vi "RTS Station 5 Doors.vi"(0 "All Door Opener Ctrl in":T11={"Station 1"={"Station Freezer"={"Time Count (s)"=0.0, "Status"="", "Door State"=FALSE, "Delay"=FALSE, "Chamber 1-1"=[], "Index"=0, "Delay Status"=""}, "Station Cab"={"Time Count (s)"=0.0, "Status"="", "Door State"=FALSE, "Delay"=FALSE, "Chamber 1-1"=[], "Index"=0, "Delay Status"=""}, "Station Slide"={"Time Count (s)"=0.0, "Status"="", "Door State"=FALSE, "Delay"=FALSE, "Chamber 1-1"=[], "Index"=0, "Delay Status"=""}, "1st Complete"=FALSE, "2nd Complete"=FALSE, "3rd Complete"=FALSE}, "Station 2"={"Station Freezer"={"Time Count (s)"=0.0, "Status"="", "Door State"=FALSE, "Delay"=FALSE, "Chamber 1-1"=[], "Index"=0, "Delay Status"=""}, "Station Cab"={"Time Count (s)"=0.0, "Status"="", "Door State"=FALSE, "Delay"=FALSE, "Chamber 1-1"=[], "Index"=0, "Delay Status"=""}, "Station Slide"={"Time Count (s)"=0.0, "Status"="", "Door State"=FALSE, "Delay"=FALSE, "Chamber 1-1"=[], "Index"=0, "Delay Status"=""}, "1st Complete"=FALSE, "2nd Complete"=FALSE, "3rd Complete"=FALSE}, "Station 3"={"Station Freezer"={"Time Count (s)"=0.0, "Status"="", "Door State"=FALSE, "Delay"=FALSE, "Chamber 1-1"=[], "Index"=0, "Delay Status"=""}, "Station Cab"={"Time Count (s)"=0.0, "Status"="", "Door State"=FALSE, "Delay"=FALSE, "Chamber 1-1"=[], "Index"=0, "Delay Status"=""}, "Station Slide"={"Time Count (s)"=0.0, "Status"="", "Door State"=FALSE, "Delay"=FALSE, "Chamber 1-1"=[], "Index"=0, "Delay Status"=""}, "1st Complete"=FALSE, "2nd Complete"=FALSE, "3rd Complete"=FALSE}, "Station 4"={"Station Freezer"={"Time Count (s)"=0.0, "Status"="", "Door State"=FALSE, "Delay"=FALSE, "Chamber 1-1"=[], "Index"=0, "Delay Status"=""}, "Station Cab"={"Time Count (s)"=0.0, "Status"="", "Door State"=FALSE, "Delay"=FALSE, "Chamber 1-1"=[], "Index"=0, "Delay Status"=""}, "Station Slide"={"Time Count (s)"=0.0, "Status"="", "Door State"=FALSE, "Delay"=FALSE, "Chamber 1-1"=[], "Index"=0, "Delay Status"=""}, "1st Complete"=FALSE, "2nd Complete"=FALSE, "3rd Complete"=FALSE}, "Station 5"={"Station Freezer"={"Time Count (s)"=0.0, "Status"="", "Door State"=FALSE, "Delay"=TRUE, "Chamber 1-1"=[], "Index"=0, "Delay Status"=""}, "Station Cab"={"Time Count (s)"=0.0, "Status"="", "Door State"=FALSE, "Delay"=TRUE, "Chamber 1-1"=[], "Index"=0, "Delay Status"=""}, "Station Slide"={"Time Count (s)"=0.0, "Status"="", "Door State"=FALSE, "Delay"=TRUE, "Chamber 1-1"=[], "Index"=0, "Delay Status"=""}, "1st Complete"=FALSE, "2nd Complete"=FALSE, "3rd Complete"=FALSE}, "Station 6"={"Station Freezer"={"Time Count (s)"=0.0, "Status"="", "Door State"=FALSE, "Delay"=TRUE, "Chamber 1-1"=[], "Index"=0, "Delay Status"=""}, "Station Cab"={"Time Count (s)"=0.0, "Status"="", "Door State"=FALSE, "Delay"=TRUE, "Chamber 1-1"=[], "Index"=0, "Delay Status"=""}, "Station Slide"={"Time Count (s)"=0.0, "Status"="", "Door State"=FALSE, "Delay"=TRUE, "Chamber 1-1"=[], "Index"=0, "Delay Status"=""}, "1st Complete"=FALSE, "2nd Complete"=FALSE, "3rd Complete"=FALSE}, "Station 7"={"Station Freezer"={"Time Count (s)"=0.0, "Status"="", "Door State"=FALSE, "Delay"=TRUE, "Chamber 1-1"=[], "Index"=0, "Delay Status"=""}, "Station Cab"={"Time Count (s)"=0.0, "Status"="", "Door State"=FALSE, "Delay"=TRUE, "Chamber 1-1"=[], "Index"=0, "Delay Status"=""}, "Station Slide"={"Time Count (s)"=0.0, "Status"="", "Door State"=FALSE, "Delay"=TRUE, "Chamber 1-1"=[], "Index"=0, "Delay Status"=""}, "1st Complete"=FALSE, "2nd Complete"=FALSE, "3rd Complete"=FALSE}, "Station 8"={"Station Freezer"={"Time Count (s)"=0.0, "Status"="", "Door State"=FALSE, "Delay"=TRUE, "Chamber 1-1"=[], "Index"=0, "Delay Status"=""}, "Station Cab"={"Time Count (s)"=0.0, "Status"="", "Door State"=FALSE, "Delay"=TRUE, "Chamber 1-1"=[], "Index"=0, "Delay Status"=""}, "Station Slide"={"Time Count (s)"=0.0, "Status"="", "Door State"=FALSE, "Delay"=TRUE, "Chamber 1-1"=[], "Index"=0, "Delay Status"=""}, "1st Complete"=FALSE, "2nd Complete"=FALSE, "3rd Complete"=FALSE}} {"Station 8"."Station Slide"."Chamber 1-1"."Start Time" format="%<%X\n%x>T"; "Station 8"."Station Slide"."Chamber 1-1"."End Time" format="%<%X\n%x>T"; "Station 8"."Station Slide"."Time Count (s)" format="%.2f"; "Station 8"."Station Cab"."Chamber 1-1"."Start Time" format="%<%X\n%x>T"; "Station 8"."Station Cab"."Chamber 1-1"."End Time" format="%<%X\n%x>T"; "Station 8"."Station Cab"."Time Count (s)" format="%.2f"; "Station 8"."Station Freezer"."Chamber 1-1"."Start Time" format="%<%X\n%x>T"; "Station 8"."Station Freezer"."Chamber 1-1"."End Time" format="%<%X\n%x>T"; "Station 8"."Station Freezer"."Time Count (s)" format="%.2f"; "Station 7"."Station Slide"."Chamber 1-1"."Start Time" format="%<%X\n%x>T"; "Station 7"."Station Slide"."Chamber 1-1"."End Time" format="%<%X\n%x>T"; "Station 7"."Station Slide"."Time Count (s)" format="%.2f"; "Station 7"."Station Cab"."Chamber 1-1"."Start Time" format="%<%X\n%x>T"; "Station 7"."Station Cab"."Chamber 1-1"."End Time" format="%<%X\n%x>T"; "Station 7"."Station Cab"."Time Count (s)" format="%.2f"; "Station 7"."Station Freezer"."Chamber 1-1"."Start Time" format="%<%X\n%x>T"; "Station 7"."Station Freezer"."Chamber 1-1"."End Time" format="%<%X\n%x>T"; "Station 7"."Station Freezer"."Time Count (s)" format="%.2f"; "Station 6"."Station Slide"."Chamber 1-1"."Start Time" format="%<%X\n%x>T"; "Station 6"."Station Slide"."Chamber 1-1"."End Time" format="%<%X\n%x>T"; "Station 6"."Station Slide"."Time Count (s)" format="%.2f"; "Station 6"."Station Cab"."Chamber 1-1"."Start Time" format="%<%X\n%x>T"; "Station 6"."Station Cab"."Chamber 1-1"."End Time" format="%<%X\n%x>T"; "Station 6"."Station Cab"."Time Count (s)" format="%.2f"; "Station 6"."Station Freezer"."Chamber 1-1"."Start Time" format="%<%X\n%x>T"; "Station 6"."Station Freezer"."Chamber 1-1"."End Time" format="%<%X\n%x>T"; "Station 6"."Station Freezer"."Time Count (s)" format="%.2f"; "Station 5"."Station Slide"."Chamber 1-1"."Start Time" format="%<%X\n%x>T"; "Station 5"."Station Slide"."Chamber 1-1"."End Time" format="%<%X\n%x>T"; "Station 5"."Station Slide"."Time Count (s)" format="%.2f"; "Station 5"."Station Cab"."Chamber 1-1"."Start Time" format="%<%X\n%x>T"; "Station 5"."Station Cab"."Chamber 1-1"."End Time" format="%<%X\n%x>T"; "Station 5"."Station Cab"."Time Count (s)" format="%.2f"; "Station 5"."Station Freezer"."Chamber 1-1"."Start Time" format="%<%X\n%x>T"; "Station 5"."Station Freezer"."Chamber 1-1"."End Time" format="%<%X\n%x>T"; "Station 5"."Station Freezer"."Time Count (s)" format="%.2f"; "Station 4"."Station Slide"."Chamber 1-1"."Start Time" format="%<%X\n%x>T"; "Station 4"."Station Slide"."Chamber 1-1"."End Time" format="%<%X\n%x>T"; "Station 4"."Station Slide"."Time Count (s)" format="%.2f"; "Station 4"."Station Cab"."Chamber 1-1"."Start Time" format="%<%X\n%x>T"; "Station 4"."Station Cab"."Chamber 1-1"."End Time" format="%<%X\n%x>T"; "Station 4"."Station Cab"."Time Count (s)" format="%.2f"; "Station 4"."Station Freezer"."Chamber 1-1"."Start Time" format="%<%X\n%x>T"; "Station 4"."Station Freezer"."Chamber 1-1"."End Time" format="%<%X\n%x>T"; "Station 4"."Station Freezer"."Time Count (s)" format="%.2f"; "Station 3"."Station Slide"."Chamber 1-1"."Start Time" format="%<%X\n%x>T"; "Station 3"."Station Slide"."Chamber 1-1"."End Time" format="%<%X\n%x>T"; "Station 3"."Station Slide"."Time Count (s)" format="%.2f"; "Station 3"."Station Cab"."Chamber 1-1"."Start Time" format="%<%X\n%x>T"; "Station 3"."Station Cab"."Chamber 1-1"."End Time" format="%<%X\n%x>T"; "Station 3"."Station Cab"."Time Count (s)" format="%.2f"; "Station 3"."Station Freezer"."Chamber 1-1"."Start Time" format="%<%X\n%x>T"; "Station 3"."Station Freezer"."Chamber 1-1"."End Time" format="%<%X\n%x>T"; "Station 3"."Station Freezer"."Time Count (s)" format="%.2f"; "Station 2"."Station Slide"."Chamber 1-1"."Start Time" format="%<%X\n%x>T"; "Station 2"."Station Slide"."Chamber 1-1"."End Time" format="%<%X\n%x>T"; "Station 2"."Station Slide"."Time Count (s)" format="%.2f"; "Station 2"."Station Cab"."Chamber 1-1"."Start Time" format="%<%X\n%x>T"; "Station 2"."Station Cab"."Chamber 1-1"."End Time" format="%<%X\n%x>T"; "Station 2"."Station Cab"."Time Count (s)" format="%.2f"; "Station 2"."Station Freezer"."Chamber 1-1"."Start Time" format="%<%X\n%x>T"; "Station 2"."Station Freezer"."Chamber 1-1"."End Time" format="%<%X\n%x>T"; "Station 2"."Station Freezer"."Time Count (s)" format="%.2f"; "Station 1"."Station Slide"."Chamber 1-1"."Start Time" format="%<%X\n%x>T"; "Station 1"."Station Slide"."Chamber 1-1"."End Time" format="%<%X\n%x>T"; "Station 1"."Station Slide"."Time Count (s)" format="%.2f"; "Station 1"."Station Cab"."Chamber 1-1"."Start Time" format="%<%X\n%x>T"; "Station 1"."Station Cab"."Chamber 1-1"."End Time" format="%<%X\n%x>T"; "Station 1"."Station Cab"."Time Count (s)" format="%.2f"; "Station 1"."Station Freezer"."Chamber 1-1"."Start Time" format="%<%X\n%x>T"; "Station 1"."Station Freezer"."Chamber 1-1"."End Time" format="%<%X\n%x>T"; "Station 1"."Station Freezer"."Time Count (s)" format="%.2f"}, 1 "Door Output Relays":T10, 5 "Input":refnum<class "Modbus Master.lvclass">, 7 "RTS Config Setup Input":T1, 11 "Error In":errorcluster) -> (4 "All Door Opener Ctrl Output":T11={"Station 1"={"Station Freezer"={"Time Count (s)"=0.0, "Status"="", "Door State"=FALSE, "Delay"=TRUE, "Chamber 1-1"=[], "Index"=0, "Delay Status"=""}, "Station Cab"={"Time Count (s)"=0.0, "Status"="", "Door State"=FALSE, "Delay"=TRUE, "Chamber 1-1"=[], "Index"=0, "Delay Status"=""}, "Station Slide"={"Time Count (s)"=0.0, "Status"="", "Door State"=FALSE, "Delay"=TRUE, "Chamber 1-1"=[], "Index"=0, "Delay Status"=""}, "1st Complete"=TRUE, "2nd Complete"=FALSE, "3rd Complete"=FALSE}, "Station 2"={"Station Freezer"={"Time Count (s)"=0.0, "Status"="", "Door State"=FALSE, "Delay"=TRUE, "Chamber 1-1"=[], "Index"=0, "Delay Status"=""}, "Station Cab"={"Time Count (s)"=0.0, "Status"="", "Door State"=FALSE, "Delay"=TRUE, "Chamber 1-1"=[], "Index"=0, "Delay Status"=""}, "Station Slide"={"Time Count (s)"=0.0, "Status"="", "Door State"=FALSE, "Delay"=TRUE, "Chamber 1-1"=[], "Index"=0, "Delay Status"=""}, "1st Complete"=TRUE, "2nd Complete"=FALSE, "3rd Complete"=FALSE}, "Station 3"={"Station Freezer"={"Time Count (s)"=0.0, "Status"="", "Door State"=FALSE, "Delay"=TRUE, "Chamber 1-1"=[], "Index"=0, "Delay Status"=""}, "Station Cab"={"Time Count (s)"=0.0, "Status"="", "Door State"=FALSE, "Delay"=TRUE, "Chamber 1-1"=[], "Index"=0, "Delay Status"=""}, "Station Slide"={"Time Count (s)"=0.0, "Status"="", "Door State"=FALSE, "Delay"=TRUE, "Chamber 1-1"=[], "Index"=0, "Delay Status"=""}, "1st Complete"=TRUE, "2nd Complete"=FALSE, "3rd Complete"=FALSE}, "Station 4"={"Station Freezer"={"Time Count (s)"=0.0, "Status"="", "Door State"=FALSE, "Delay"=TRUE, "Chamber 1-1"=[], "Index"=0, "Delay Status"=""}, "Station Cab"={"Time Count (s)"=0.0, "Status"="", "Door State"=FALSE, "Delay"=TRUE, "Chamber 1-1"=[], "Index"=0, "Delay Status"=""}, "Station Slide"={"Time Count (s)"=0.0, "Status"="", "Door State"=FALSE, "Delay"=TRUE, "Chamber 1-1"=[], "Index"=0, "Delay Status"=""}, "1st Complete"=TRUE, "2nd Complete"=FALSE, "3rd Complete"=FALSE}, "Station 5"={"Station Freezer"={"Time Count (s)"=0.0, "Status"="", "Door State"=TRUE, "Delay"=TRUE, "Chamber 1-1"=[], "Index"=0, "Delay Status"=""}, "Station Cab"={"Time Count (s)"=0.0, "Status"="", "Door State"=FALSE, "Delay"=TRUE, "Chamber 1-1"=[], "Index"=0, "Delay Status"=""}, "Station Slide"={"Time Count (s)"=0.0, "Status"="", "Door State"=FALSE, "Delay"=TRUE, "Chamber 1-1"=[], "Index"=0, "Delay Status"=""}, "1st Complete"=TRUE, "2nd Complete"=FALSE, "3rd Complete"=FALSE}, "Station 6"={"Station Freezer"={"Time Count (s)"=0.0, "Status"="", "Door State"=FALSE, "Delay"=TRUE, "Chamber 1-1"=[], "Index"=0, "Delay Status"=""}, "Station Cab"={"Time Count (s)"=0.0, "Status"="", "Door State"=FALSE, "Delay"=TRUE, "Chamber 1-1"=[], "Index"=0, "Delay Status"=""}, "Station Slide"={"Time Count (s)"=0.0, "Status"="", "Door State"=FALSE, "Delay"=TRUE, "Chamber 1-1"=[], "Index"=0, "Delay Status"=""}, "1st Complete"=TRUE, "2nd Complete"=FALSE, "3rd Complete"=FALSE}, "Station 7"={"Station Freezer"={"Time Count (s)"=0.0, "Status"="", "Door State"=FALSE, "Delay"=TRUE, "Chamber 1-1"=[], "Index"=0, "Delay Status"=""}, "Station Cab"={"Time Count (s)"=0.0, "Status"="", "Door State"=FALSE, "Delay"=TRUE, "Chamber 1-1"=[], "Index"=0, "Delay Status"=""}, "Station Slide"={"Time Count (s)"=0.0, "Status"="", "Door State"=FALSE, "Delay"=TRUE, "Chamber 1-1"=[], "Index"=0, "Delay Status"=""}, "1st Complete"=TRUE, "2nd Complete"=FALSE, "3rd Complete"=FALSE}, "Station 8"={"Station Freezer"={"Time Count (s)"=0.0, "Status"="", "Door State"=FALSE, "Delay"=TRUE, "Chamber 1-1"=[], "Index"=0, "Delay Status"=""}, "Station Cab"={"Time Count (s)"=0.0, "Status"="", "Door State"=FALSE, "Delay"=TRUE, "Chamber 1-1"=[], "Index"=0, "Delay Status"=""}, "Station Slide"={"Time Count (s)"=0.0, "Status"="", "Door State"=FALSE, "Delay"=TRUE, "Chamber 1-1"=[], "Index"=0, "Delay Status"=""}, "1st Complete"=TRUE, "2nd Complete"=FALSE, "3rd Complete"=FALSE}} {"Station 8"."Station Slide"."Chamber 1-1"."Start Time" format="%<%X\n%x>T"; "Station 8"."Station Slide"."Chamber 1-1"."End Time" format="%<%X\n%x>T"; "Station 8"."Station Slide"."Time Count (s)" format="%.2f"; "Station 8"."Station Cab"."Chamber 1-1"."Start Time" format="%<%X\n%x>T"; "Station 8"."Station Cab"."Chamber 1-1"."End Time" format="%<%X\n%x>T"; "Station 8"."Station Cab"."Time Count (s)" format="%.2f"; "Station 8"."Station Freezer"."Chamber 1-1"."Start Time" format="%<%X\n%x>T"; "Station 8"."Station Freezer"."Chamber 1-1"."End Time" format="%<%X\n%x>T"; "Station 8"."Station Freezer"."Time Count (s)" format="%.2f"; "Station 7"."Station Slide"."Chamber 1-1"."Start Time" format="%<%X\n%x>T"; "Station 7"."Station Slide"."Chamber 1-1"."End Time" format="%<%X\n%x>T"; "Station 7"."Station Slide"."Time Count (s)" format="%.2f"; "Station 7"."Station Cab"."Chamber 1-1"."Start Time" format="%<%X\n%x>T"; "Station 7"."Station Cab"."Chamber 1-1"."End Time" format="%<%X\n%x>T"; "Station 7"."Station Cab"."Time Count (s)" format="%.2f"; "Station 7"."Station Freezer"."Chamber 1-1"."Start Time" format="%<%X\n%x>T"; "Station 7"."Station Freezer"."Chamber 1-1"."End Time" format="%<%X\n%x>T"; "Station 7"."Station Freezer"."Time Count (s)" format="%.2f"; "Station 6"."Station Slide"."Chamber 1-1"."Start Time" format="%<%X\n%x>T"; "Station 6"."Station Slide"."Chamber 1-1"."End Time" format="%<%X\n%x>T"; "Station 6"."Station Slide"."Time Count (s)" format="%.2f"; "Station 6"."Station Cab"."Chamber 1-1"."Start Time" format="%<%X\n%x>T"; "Station 6"."Station Cab"."Chamber 1-1"."End Time" format="%<%X\n%x>T"; "Station 6"."Station Cab"."Time Count (s)" format="%.2f"; "Station 6"."Station Freezer"."Chamber 1-1"."Start Time" format="%<%X\n%x>T"; "Station 6"."Station Freezer"."Chamber 1-1"."End Time" format="%<%X\n%x>T"; "Station 6"."Station Freezer"."Time Count (s)" format="%.2f"; "Station 5"."Station Slide"."Chamber 1-1"."Start Time" format="%<%X\n%x>T"; "Station 5"."Station Slide"."Chamber 1-1"."End Time" format="%<%X\n%x>T"; "Station 5"."Station Slide"."Time Count (s)" format="%.2f"; "Station 5"."Station Cab"."Chamber 1-1"."Start Time" format="%<%X\n%x>T"; "Station 5"."Station Cab"."Chamber 1-1"."End Time" format="%<%X\n%x>T"; "Station 5"."Station Cab"."Time Count (s)" format="%.2f"; "Station 5"."Station Freezer"."Chamber 1-1"."Start Time" format="%<%X\n%x>T"; "Station 5"."Station Freezer"."Chamber 1-1"."End Time" format="%<%X\n%x>T"; "Station 5"."Station Freezer"."Time Count (s)" format="%.2f"; "Station 4"."Station Slide"."Chamber 1-1"."Start Time" format="%<%X\n%x>T"; "Station 4"."Station Slide"."Chamber 1-1"."End Time" format="%<%X\n%x>T"; "Station 4"."Station Slide"."Time Count (s)" format="%.2f"; "Station 4"."Station Cab"."Chamber 1-1"."Start Time" format="%<%X\n%x>T"; "Station 4"."Station Cab"."Chamber 1-1"."End Time" format="%<%X\n%x>T"; "Station 4"."Station Cab"."Time Count (s)" format="%.2f"; "Station 4"."Station Freezer"."Chamber 1-1"."Start Time" format="%<%X\n%x>T"; "Station 4"."Station Freezer"."Chamber 1-1"."End Time" format="%<%X\n%x>T"; "Station 4"."Station Freezer"."Time Count (s)" format="%.2f"; "Station 3"."Station Slide"."Chamber 1-1"."Start Time" format="%<%X\n%x>T"; "Station 3"."Station Slide"."Chamber 1-1"."End Time" format="%<%X\n%x>T"; "Station 3"."Station Slide"."Time Count (s)" format="%.2f"; "Station 3"."Station Cab"."Chamber 1-1"."Start Time" format="%<%X\n%x>T"; "Station 3"."Station Cab"."Chamber 1-1"."End Time" format="%<%X\n%x>T"; "Station 3"."Station Cab"."Time Count (s)" format="%.2f"; "Station 3"."Station Freezer"."Chamber 1-1"."Start Time" format="%<%X\n%x>T"; "Station 3"."Station Freezer"."Chamber 1-1"."End Time" format="%<%X\n%x>T"; "Station 3"."Station Freezer"."Time Count (s)" format="%.2f"; "Station 2"."Station Slide"."Chamber 1-1"."Start Time" format="%<%X\n%x>T"; "Station 2"."Station Slide"."Chamber 1-1"."End Time" format="%<%X\n%x>T"; "Station 2"."Station Slide"."Time Count (s)" format="%.2f"; "Station 2"."Station Cab"."Chamber 1-1"."Start Time" format="%<%X\n%x>T"; "Station 2"."Station Cab"."Chamber 1-1"."End Time" format="%<%X\n%x>T"; "Station 2"."Station Cab"."Time Count (s)" format="%.2f"; "Station 2"."Station Freezer"."Chamber 1-1"."Start Time" format="%<%X\n%x>T"; "Station 2"."Station Freezer"."Chamber 1-1"."End Time" format="%<%X\n%x>T"; "Station 2"."Station Freezer"."Time Count (s)" format="%.2f"; "Station 1"."Station Slide"."Chamber 1-1"."Start Time" format="%<%X\n%x>T"; "Station 1"."Station Slide"."Chamber 1-1"."End Time" format="%<%X\n%x>T"; "Station 1"."Station Slide"."Time Count (s)" format="%.2f"; "Station 1"."Station Cab"."Chamber 1-1"."Start Time" format="%<%X\n%x>T"; "Station 1"."Station Cab"."Chamber 1-1"."End Time" format="%<%X\n%x>T"; "Station 1"."Station Cab"."Time Count (s)" format="%.2f"; "Station 1"."Station Freezer"."Chamber 1-1"."Start Time" format="%<%X\n%x>T"; "Station 1"."Station Freezer"."Chamber 1-1"."End Time" format="%<%X\n%x>T"; "Station 1"."Station Freezer"."Time Count (s)" format="%.2f"}, 6 "Output":refnum<class "Modbus Master.lvclass">, 8 "RTS Config Setup Output":T1, 10 "States":string, 15 "Error Out":errorcluster)   [LabVIEW 2016]
uses:
  Type Definitions/RTS All Station Door Opener Ctrl.ctl
  Type Definitions/RTS Station Relay Ops.ctl
  Type Definitions/RTS Door Opener Indicator.ctl
  Type Definitions/RTS Door Ops Client.ctl
  Type Definitions/RTS Door Opening Schedule.ctl
  Type Definitions/RTS Door Ops Sequence.ctl
  <vilib>/NI/Modbus Library/API/Master/Modbus Master.lvclass
  Drivers/WAGO 750-881/Type Definitions/Wago Door Relays.ctl
  Type Definitions/RTS Configuration Setup.ctl
  Type Definitions/RTS Wago Config.ctl
  Type Definitions/RTS APLUS Config.ctl
  Type Definitions/RTS Yokogawa MX Config.ctl
  Type Definitions/RTS Replay Server Control.ctl
  Type Definitions/RTS Server Configuration.ctl
  Type Definitions/RTS Station Settions TCP Comms.ctl
  Type Definitions/RTS Chamber Save Status.ctl
  Type Definitions/RTS Test Pattern.ctl
panel:
  # "Chamber Conditions:"
  # "Chamber Conditions:"
  # "Chamber Conditions:"
  # "Chamber Conditions:"
  # "Chamber Conditions:"
  # "Chamber Conditions:"
  # "Chamber Conditions:"
  # "Chamber Conditions:"
  # "Chamber Conditions:"
  # "Chamber Conditions:"
  # "Chamber Conditions:"
  # "Chamber Conditions:"
  # "Chamber Conditions:"
  # "Chamber Conditions:"
  # "Chamber Conditions:"
  # "Chamber Conditions:"
  # "Chamber Conditions:"
  # "Chamber Conditions:"
  # "Chamber Conditions:"
  # "Chamber Conditions:"
  # "Chamber Conditions:"
  # "Chamber Conditions:"
  # "Chamber Conditions:"
  # "Chamber Conditions:"
  # "Chamber Conditions:"
  # "Chamber Conditions:"
  # "Chamber Conditions:"
  # "Chamber Conditions:"
  # "Chamber Conditions:"
  # "Chamber Conditions:"
  # "Chamber Conditions:"
  # "Chamber Conditions:"
  # "Chamber Conditions:"
  # "Chamber Conditions:"
  # "Chamber Conditions:"
  # "Chamber Conditions:"
  # "Chamber Conditions:"
  # "Chamber Conditions:"
  # "Chamber Conditions:"
  # "Chamber Conditions:"
  # "Chamber Conditions:"
  # "Chamber Conditions:"
  # "Chamber Conditions:"
  # "Chamber Conditions:"
  # "Chamber Conditions:"
  # "Chamber Conditions:"
  # "Chamber Conditions:"
  # "Chamber Conditions:"
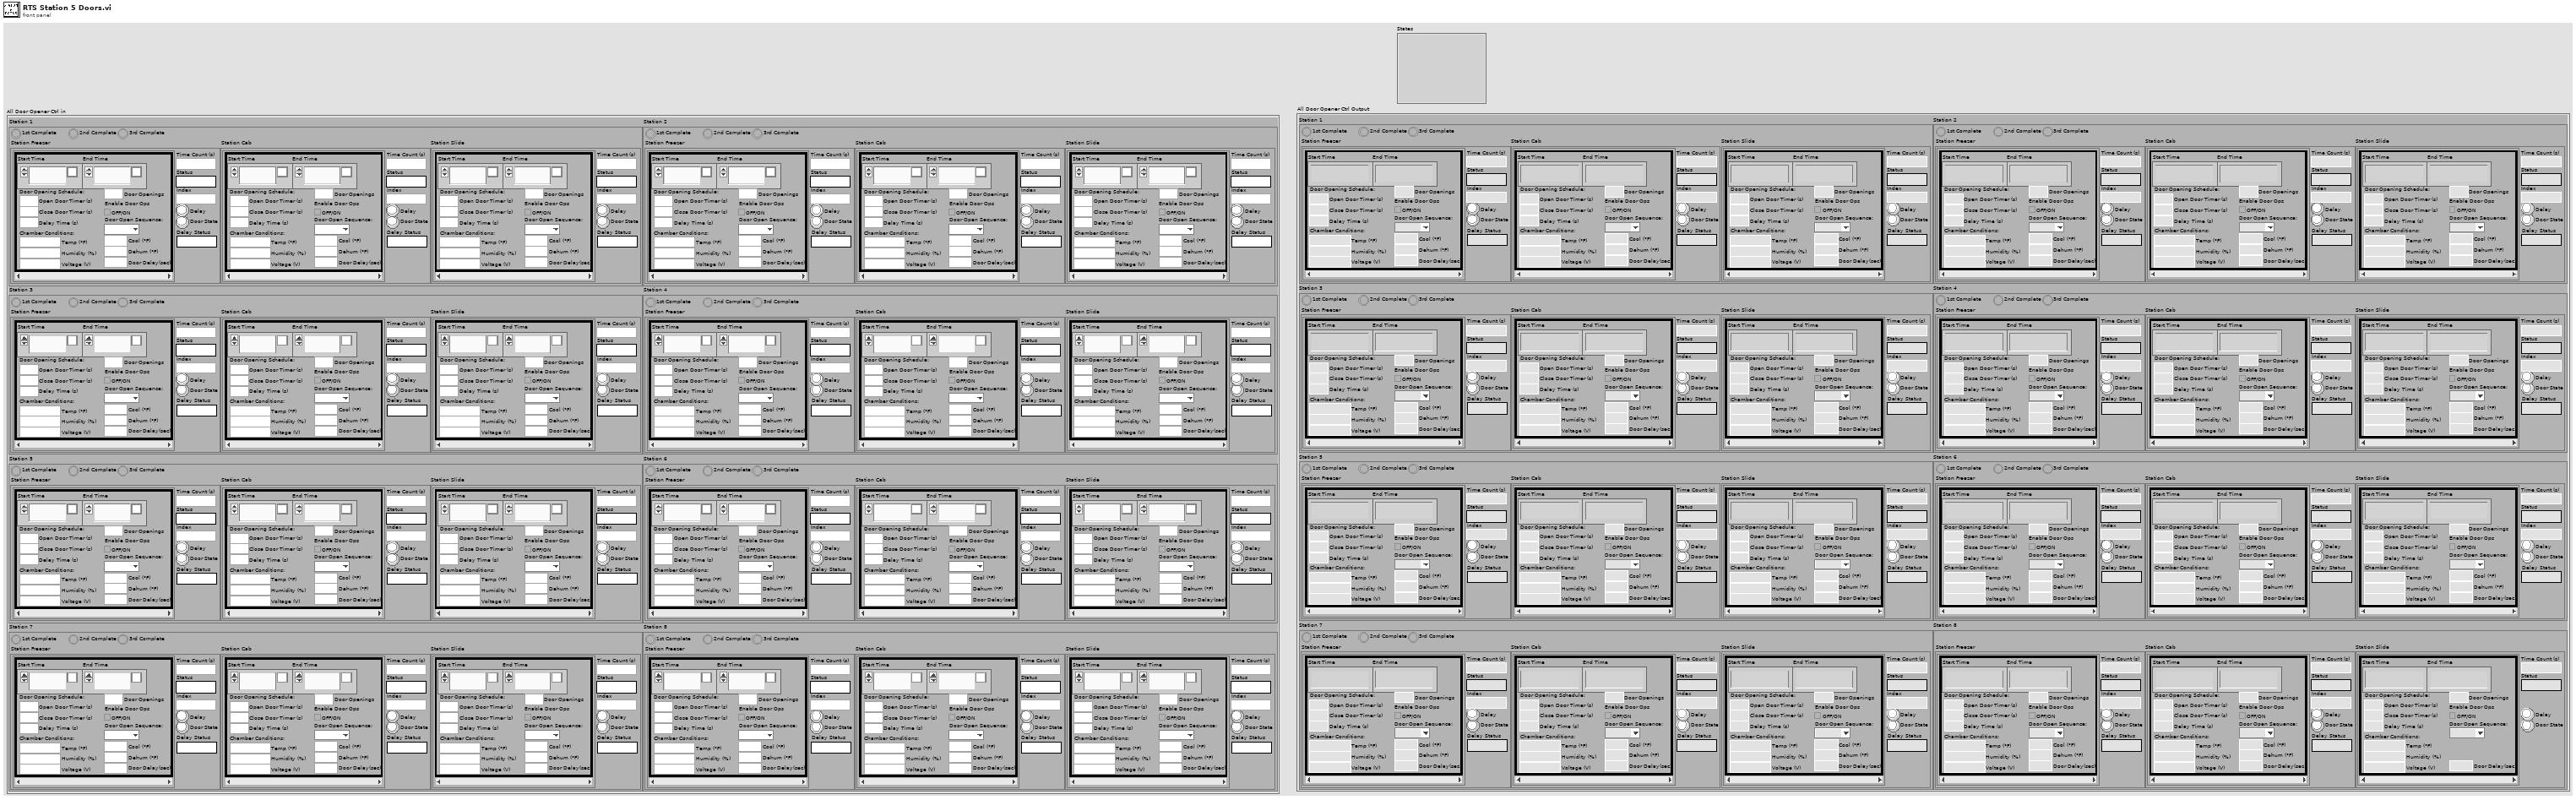
[diagram p1: front panel]
types:
  T1 = typedef "RTS Configuration Setup.ctl" = cluster{"Wago RTS":T2, "APLUS Array":T3[], "Yokogawa MX100 RTS Array":T4[], "Replay Server":T5[], "Server Configuration Array":T6[], "Station Settings":T7}
  T2 = typedef "RTS Wago Config.ctl" = cluster{"Disable":u16, "Interval":u16, "Controller":u16, "Address":u16, "IP Address":string, "AtoDmax":u16, "FullScale":u16, "VoltageType":u16, "Window1":u16, "Control1":u16, "Window2":u16, "Control2":u16}
  T3 = typedef "RTS APLUS Config.ctl" = cluster{"Disable":u16, "IP Address":string, "Input (4 Wire Unbalanced Load)":u16, "Dual Input (L1 115V, L2 230V)":u16, "LowLeakLimit":dbl, "Voltage Type":u16}
  T4 = typedef "RTS Yokogawa MX Config.ctl" = cluster{"IP Address":string, "TC Type":string, "Interval":u16, "Single Range":u16, "CalcWh":u16}
  T5 = typedef "RTS Replay Server Control.ctl" = cluster{"Interval":i16, "Repeat":u16, "Station":u16, "Load Path":path, "AutoMap":u16, "WattFactor":dbl, "AmpFactor":dbl}
  T6 = typedef "RTS Server Configuration.ctl" = cluster{"System":u16, "SysID":u16, "Title":string, "Enabled Server":u16, "Directory":string, "Configuration":string, "ValUpdate":u16, "TrendUpdate":u16, "ControlUpdate":u16, "Monitor":u16, "Pfact":u16, "Pipe":string, "TcpIP":u16, "Tunit":string, "ResultPath":path, "Door Sch DataLink":path, "MaxTCRate":u16, "Recovery":u16, "AutoRecovery":u16, "UsePowerFactor":u16, "OperatorPath":string, "Room":u16, "Station":u16, "Title":string, "DefMake":string, "Enabled Stall":u16, "Room":u16, "Title":string, "Station 1":u16, "Enabled 1":u16, "Station 2":u16, "Enabled 2":u16, "Station 3":u16, "Enabled 3":u16, "Station 4":u16, "Enabled 4":u16, "Station 5":u16, "Enabled 5":u16, "Station 6":u16, "Enabled 6":u16, "Station 7":u16, "Enabled 7":u16, "Station 8":u16, "Enabled 8":u16, "Title S1":string, "Title S2":string, "Title S3":string, "Title S5":string, "Title S6":string, "Title S7":string, "Title S8":string, "Title S4":string}
  T7 = typedef "RTS Station Settions TCP Comms.ctl" = cluster{"Point Files":cluster{"Point File 1":path, "Point File 2":path, "Point File 3":path, "Point File 4":path, "Point File 5":path, "Point File 6":path, "Point File 7":path, "Point File 8":path}, "Save Status":T8, "Setup Info":cluster{"Setup Info Station 1":string[][], "Setup Info Station 2":string[][], "Setup Info Station 3":string[][], "Setup Info Station 4":string[][], "Setup Info Station 5":string[][], "Setup Info Station 6":string[][], "Setup Info Station 7":string[][], "Setup Info Station 8":string[][]}, "Chamber Test Pattern":T9}
  T8 = typedef "RTS Chamber Save Status.ctl" = cluster{"Save Status 1":bool, "Save Status 2":bool, "Save Status 3":bool, "Save Status 4":bool, "Save Status 5":bool, "Save Status 6":bool, "Save Status 7":bool, "Save Status 8":bool}
  T9 = typedef "RTS Test Pattern.ctl" = cluster{" Pattern 1":path, "Pattern 2":path, "Pattern 3":path, "Pattern 4":path, "Pattern 5":path, "Pattern 6":path, "Pattern 7":path, "Pattern 8":path}
  T10 = typedef "Wago Door Relays.ctl" = cluster{"Station 1 Freezer":bool, "Station 1 Cab":bool, "Station 1 Slide":bool, "Station 2 Freezer":bool, "Station 2 Cab":bool, "Station 2 Slide":bool, "Station 3 Freezer":bool, "Station 3 Cab":bool, "Station 3 Slide":bool, "Station 4 Freezer":bool, "Station 4 Cab":bool, "Station 4 Slide":bool, "Station 5 Freezer":bool, "Station 5 Cab":bool, "Station 5 Slide":bool, "Station 6 Freezer":bool, "Station 6 Cab":bool, "Station 6 Slide":bool, "Station 7 Freezer":bool, "Station 7 Cab":bool, "Station 7 Slide":bool, "Station 8 Freezer":bool, "Station 8 Cab":bool, "Station 8 Slide":bool, "Door Opener Enable":bool}
  T11 = typedef "RTS All Station Door Opener Ctrl.ctl" = cluster{"Station 1":T12, "Station 2":T12, "Station 3":T12, "Station 4":T12, "Station 5":T12, "Station 6":T12, "Station 7":T12, "Station 8":T12}
  T12 = typedef "RTS Station Relay Ops.ctl" = cluster{"Station Freezer":T13, "Station Cab":T13, "Station Slide":T13, "1st Complete":bool, "2nd Complete":bool, "3rd Complete":bool}
  T13 = typedef "RTS Door Opener Indicator.ctl" = cluster{"Time Count (s)":dbl, "Status":string, "Door State":bool, "Delay":bool, "Chamber 1-1":T14[], "Index":i32, "Delay Status":string}
  T14 = typedef "RTS Door Ops Client.ctl" = cluster{"End Time":timestamp, "Start Time":timestamp, "Door Opening Schedule:":T15, "Enable Door Ops":bool, "Door Openings":u32, "Temp (°F)":dbl, "Humidity (%)":dbl, "Voltage (V)":dbl, "Door Open Sequence:":T16, "Door Delay(sec)":dbl, "Dehum (°F)":dbl, "Cool (°F)":dbl}
  T15 = typedef "RTS Door Opening Schedule.ctl" = cluster{"Open Door Timer (s)":dbl, "Delay Time (s)":dbl, "Close Door Timer (s)":dbl}
  T16 = typedef "RTS Door Ops Sequence.ctl" = enum16{"", "1st", "2nd", "3rd"}
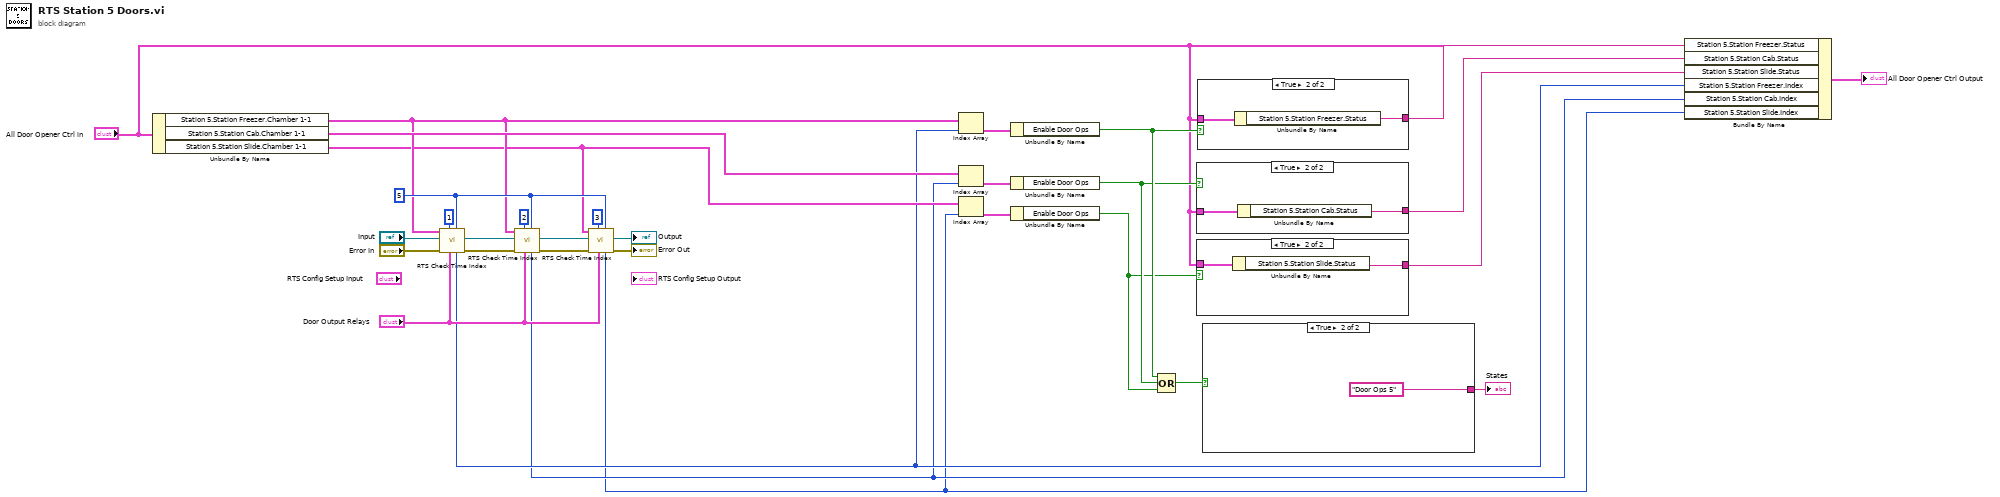
[diagram p0: block diagram]
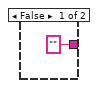
[diagram p2: hidden frame]
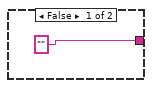
[diagram p3: hidden frame]
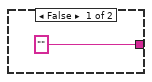
[diagram p4: hidden frame]
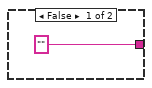
[diagram p5: hidden frame]
diagram:
  w18 = u8 5 ("Station #")
  n1 = Unbundle By Name("All Door Opener Ctrl in") -> ("Station 5.Station Freezer.Chamber 1-1"=w10:T14[], "Station 5.Station Cab.Chamber 1-1"=w27:T14[], "Station 5.Station Slide.Chamber 1-1"=w9:T14[])
  n2 = call "RTS Check Time Index.vi"("Station #"=w18, "Door Output Relays"="Door Output Relays", "Relay #"=u8 1, "Error In"="Error In", "Input"="Input", "Chamber 1-1 Input"=w10) -> ("Error Out"=w11:errorcluster, "Output"=w13:refnum<class "Modbus Master.lvclass">, "Index Number"=w3:i32)  [unwired: 2 in, 1 out]
  n3 = call "RTS Check Time Index.vi"("Station #"=w18, "Door Output Relays"="Door Output Relays", "Relay #"=u8 2, "Error In"=w11, "Input"=w13, "Chamber 1-1 Input"=w10) -> ("Error Out"=w12:errorcluster, "Output"=w14:refnum<class "Modbus Master.lvclass">, "Index Number"=w2:i32)  [unwired: 2 in, 1 out]
  n4 = call "RTS Check Time Index.vi"("Station #"=w18, "Door Output Relays"="Door Output Relays", "Relay #"=u8 3, "Error In"=w12, "Input"=w14, "Chamber 1-1 Input"=w9) -> ("Error Out"=→"Error Out":errorcluster, "Output"=→"Output":refnum<class "Modbus Master.lvclass">, "Index Number"=w1:i32)  [unwired: 2 in, 1 out]
  n5 = Index Array(array=w10, index=w3) -> (element=w28:T14)
  n6 = Index Array(array=w27, index=w2) -> (element=w30:T14)
  n7 = Index Array(array=w9, index=w1) -> (element=w29:T14)
  n8 = Unbundle By Name(w28) -> ("Enable Door Ops"=w26:bool)
  n9 = Unbundle By Name(w30) -> ("Enable Door Ops"=w25:bool)
  n10 = Unbundle By Name(w29) -> ("Enable Door Ops"=w24:bool)
  n11 = Compound Arithmetic op=OR(w26, w25, w24) -> (w31:bool)
  n12 = case shown="True" w25 {
    tunnel: ["" w34] -> w21
    tunnel: "All Door Opener Ctrl in" -> [_ w35]
    frame False {
    }
    frame True {
      n13 = Unbundle By Name(w35) -> ("Station 5.Station Cab.Status"=w34:string)
    }
  }
  n14 = case shown="True" w24 {
    tunnel: ["" w37] -> w20
    tunnel: "All Door Opener Ctrl in" -> [_ w38]
    frame False {
    }
    frame True {
      n15 = Unbundle By Name(w38) -> ("Station 5.Station Slide.Status"=w37:string)
    }
  }
  n16 = case shown="True" w26 {
    tunnel: ["" w40] -> w23
    tunnel: "All Door Opener Ctrl in" -> [_ w41]
    frame False {
    }
    frame True {
      n17 = Unbundle By Name(w41) -> ("Station 5.Station Freezer.Status"=w40:string)
    }
  }
  n18 = case shown="True" w31 {
    tunnel: ["" ("State(s) in Front (\"\")") "Door Ops 5" ("State(s) in Front (\"\")")] -> w32
    frame False {
    }
    frame True {
    }
  }
  "States" <- w32
  n19 = Bundle By Name(cluster="All Door Opener Ctrl in", "Station 5.Station Freezer.Status"=w23, "Station 5.Station Cab.Status"=w21, "Station 5.Station Slide.Status"=w20, "Station 5.Station Freezer.Index"=w3, "Station 5.Station Cab.Index"=w2, "Station 5.Station Slide.Index"=w1) -> (→"All Door Opener Ctrl Output":T11)
